vi "TestObservePath_ValueCFolderFileDotExt.vi"(8 "error in (no error)":errorcluster, 11 "TestCase in":refnum<class "TestObservableDataTypes.lvclass">) -> (0 "error out":errorcluster, 3 "TestCase out":refnum<class "TestObservableDataTypes.lvclass">)   [LabVIEW 2017, in "TestObservableDataTypes.lvclass"]
uses:
  TestObservableDataTypes.lvclass
  Source/Framework/IMediator/IMediator Messages/Subscribe Msg/Subscribe Msg.lvclass
  Source/Framework/IMediator/SubscriptionRequest/SubscriptionRequest.lvclass
  Source/Framework/IMediator/ISubscriptionPolicy/ISubscriptionPolicy.lvclass
  Source/Framework/SubscriptionPolicy/BasicSubscription/BasicSubscription.lvclass
  C:/Git/mva-framework/Source/Framework/IMediator/ISubscriptionPolicy/ISubscriptionPolicy.lvclass
  gpm_packages/@cs/transport/Source/ITransport/ITransport.lvclass
panel:
  out "ControlTerminal":path
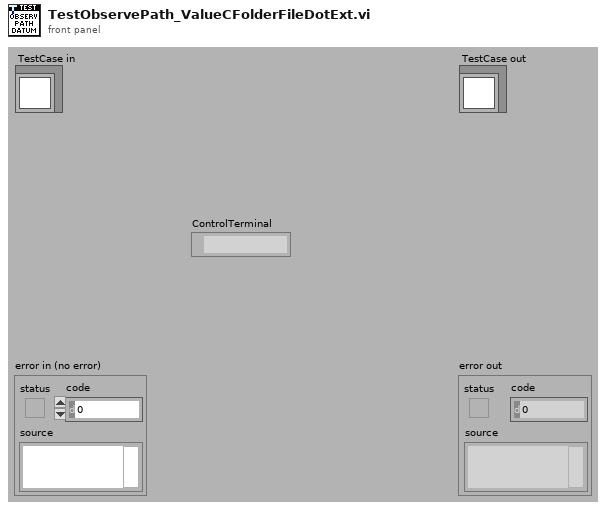
[diagram p1: front panel]
types:
  T1 = typedef "IMediator.lvlib/ISubscriptionPolicy.lvclass/ISubscriptionPolicy Reference.ctl" = refnum<data-value>
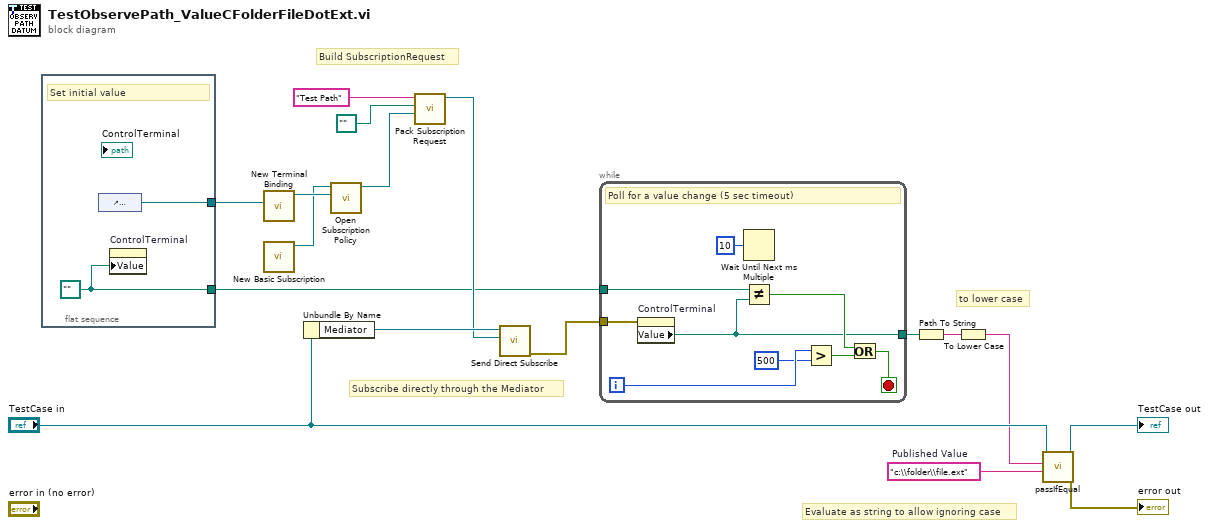
[diagram p0: block diagram]
diagram:
  w5 = "c:\\folder\\file.ext"  # Published Value
  # "to lower case"
  # "Evaluate as string to allow ignoring case"
  # "Build SubscriptionRequest"
  # "Subscribe directly through the Mediator"
  n1 = flat-sequence {
    tunnel: [w19] -> w9
    tunnel: [w18] -> w7
    frame #0 {
      w18 = path "" ("ControlTerminal")
      # "Set initial value"
      n2 = control-ref of="ControlTerminal"() -> (w19:refnum<vi>)
      n3 = property on="ControlTerminal" class="Path"("Value"=w18) -> ()  [unwired: 2 in, 2 out]
    }
  }
  n4 = call "New Terminal Binding.vi"("Ctl Refnum"=w9) -> ("TerminalBinding"=w10:refnum<class "TerminalBinding.lvclass">)  [unwired: 9 in, 1 out]
  n5 = call "New Basic Subscription.vi"() -> ("BasicSubscription Out"=w2:refnum<class "BasicSubscription.lvclass">)  [unwired: 11 in]
  n6 = Unbundle By Name("TestCase in") -> ("Mediator"=w14:refnum<class "Message Enqueuer.lvclass">)
  n7 = call "Open Subscription Policy.vi"("Transport"=w10, "SubscriptionPolicy"=w2) -> ("Subscription Policy"=w1:T1)  [unwired: 8 in, 1 out]
  n8 = call "Pack Subscription Request.vi"("Subscription Policy"=w1, "Type"=path "", "Datum Name"="Test Path" ("Topic Name")) -> ("SubscriptionRequest"=w13:refnum<class "SubscriptionRequest.lvclass">)  [unwired: 8 in]
  n9 = call "Send Direct Subscribe.vi"("Subscription Request"=w13, "Message Enqueuer"=w14) -> ("error out"=w8:errorcluster)  [unwired: 8 in, 1 out]
  n10 = while {
    tunnel: w8 -> [w28]
    tunnel: w7 -> [w27]
    tunnel: [w20] -> w6
    i -> [w23]
    stop <- w21 stop-if-true
    # "Poll for a value change (5 sec timeout)"
    n11 = property on="ControlTerminal" class="Path"(error in=w28) -> ("Value"=w20:path)  [unwired: 1 in, 2 out]
    n12 = Wait Until Next ms Multiple(millisecond multiple=u32 10 ("milliseconds to wait")) -> ()  [unwired: 1 out]
    n13 = Not Equal?(x=w27, y=w20) -> (x != y?=w26:bool)
    n14 = Greater?(x=w23, y=500) -> (0:w24:bool)
    n15 = Or(x=w26, y=w24) -> (x .or. y?=w21:bool)
  }
  n16 = Path To String(path=w6) -> (string=w4:string)
  n17 = To Lower Case(string=w4) -> (all lower case string=w3:string)
  n18 = call-dynamic "passIfEqual.vi"("y"=w5, "x"=w3, "TestCase in"="TestCase in") -> ("error out"=→"error out":errorcluster, "TestCase out"=→"TestCase out":refnum<class "TestObservableDataTypes.lvclass">)  [unwired: 7 in]
